vi "Test_Ping.vi"() -> ()   [LabVIEW 2013]
panel:
  out "Test DB?":bool=TRUE
  out "Time for ping (s)":dbl
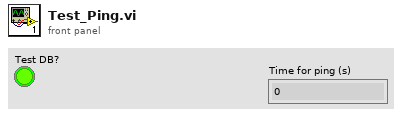
[diagram p1: front panel]
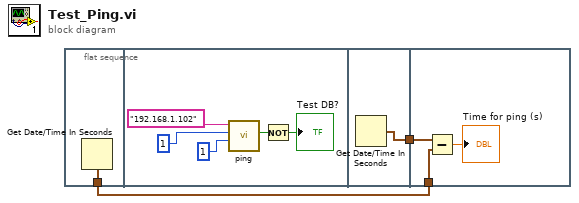
[diagram p0: block diagram]
diagram:
  n1 = flat-sequence {
    tunnel: [w3] -> w1
    tunnel: [w9] -> w2
    tunnel: w2 -> [w11]
    tunnel: w1 -> [w10]
    frame #0 {
      n2 = Get Date/Time In Seconds() -> (seconds since 1Jan1904=w3:timestamp)
    }
    frame #1 {
      n3 = call "ping.vi"("timeout (ms)"=1, "count"=1, "host"="192.168.1.102") -> ("found?"=w5:bool)  [unwired: 6 in, 2 out]
      n4 = Not(x=w5) -> (.not. x?=→"Test DB?":bool)
    }
    frame #2 {
      n5 = Get Date/Time In Seconds() -> (seconds since 1Jan1904=w9:timestamp)
    }
    frame #3 {
      n6 = Subtract(x=w11, y=w10) -> (x-y=→"Time for ping (s)":dbl)
    }
  }
